vi "Corrupt Frame.vi"(6 "Frame Infos Array":T3[](array[typedef]) {"CRC Index" min=-7 max=7; "DLC Length  Corruption Index" min=-8 max=8}, 8 "error in (no error)":errorcluster, 9 "Engine Run-Time Data Cluster In":T5 {"Compiled Data"."Corruption Info DUT_Network"."Frame Infos Array"."CRC Index" min=-7 max=7; "Compiled Data"."Corruption Info DUT_Network"."Frame Infos Array"."DLC Length  Corruption Index" min=-8 max=8; "Compiled Data"."Corruption Info Network_DUT"."Frame Infos Array"."CRC Index" min=-7 max=7; "Compiled Data"."Corruption Info Network_DUT"."Frame Infos Array"."DLC Length  Corruption Index" min=-8 max=8; "Specified Channel Ref List Out" format="%.0x"; "Specified Channel Ref List In" format="%.0x"}, 10 "Corrupt IDs Array":u32[](array[numeric]), 11 "CAN frame":T1 {"payload" format="%x"; "timestamp" format="%<%.7X\n%x>T"; "type" items=["CAN Data"=0, "CAN Remote"=1, "CAN Bus Error"=2, "CAN 2.0 Data"=8, "CAN FD Data"=16, "CAN FD+BRS Data"=24, "J1939 Data"=192, "Delay"=224, "Log Trigger"=225, "Start Trigger"=226]; "identifier" format="%x"}) -> (0 "error out":errorcluster, 2 "Disable Frame":bool, 3 "Frame Data":T1 {"payload" format="%x"; "timestamp" format="%<%.7X\n%x>T"; "type" items=["CAN Data"=0, "CAN Remote"=1, "CAN Bus Error"=2, "CAN 2.0 Data"=8, "CAN FD Data"=16, "CAN FD+BRS Data"=24, "J1939 Data"=192, "Delay"=224, "Log Trigger"=225, "Start Trigger"=226]; "identifier" format="%x"})   [LabVIEW 2018, in "CAN Gateway Engine.lvlib"]
uses:
  CAN Gateway Engine.lvlib
  <vilib>/xnet/xnet.llb/XNET Frame CAN.ctl
  <vilib>/xnet/xnet.llb/XNET Frame Type CAN.ctl
  Shared/CTLs/Runtime engine Data.ctl
  <vilib>/NI Veristand/Custom Device API/Custom Device Engine Event Ref.ctl
  <vilib>/NI Veristand/Custom Device API/Custom Device Item Ref.ctl
  Shared/CTLs/Compiled Data.ctl
  Shared/CTLs/Corruption Info.ctl
  Shared/CTLs/Frame.ctl
  Shared/CTLs/Signal_Data_Trigger.ctl
  <vilib>/NI Veristand/Custom Device API/Custom Device API.lvlib
  Shared/CAN Gateway Shared.lvlib
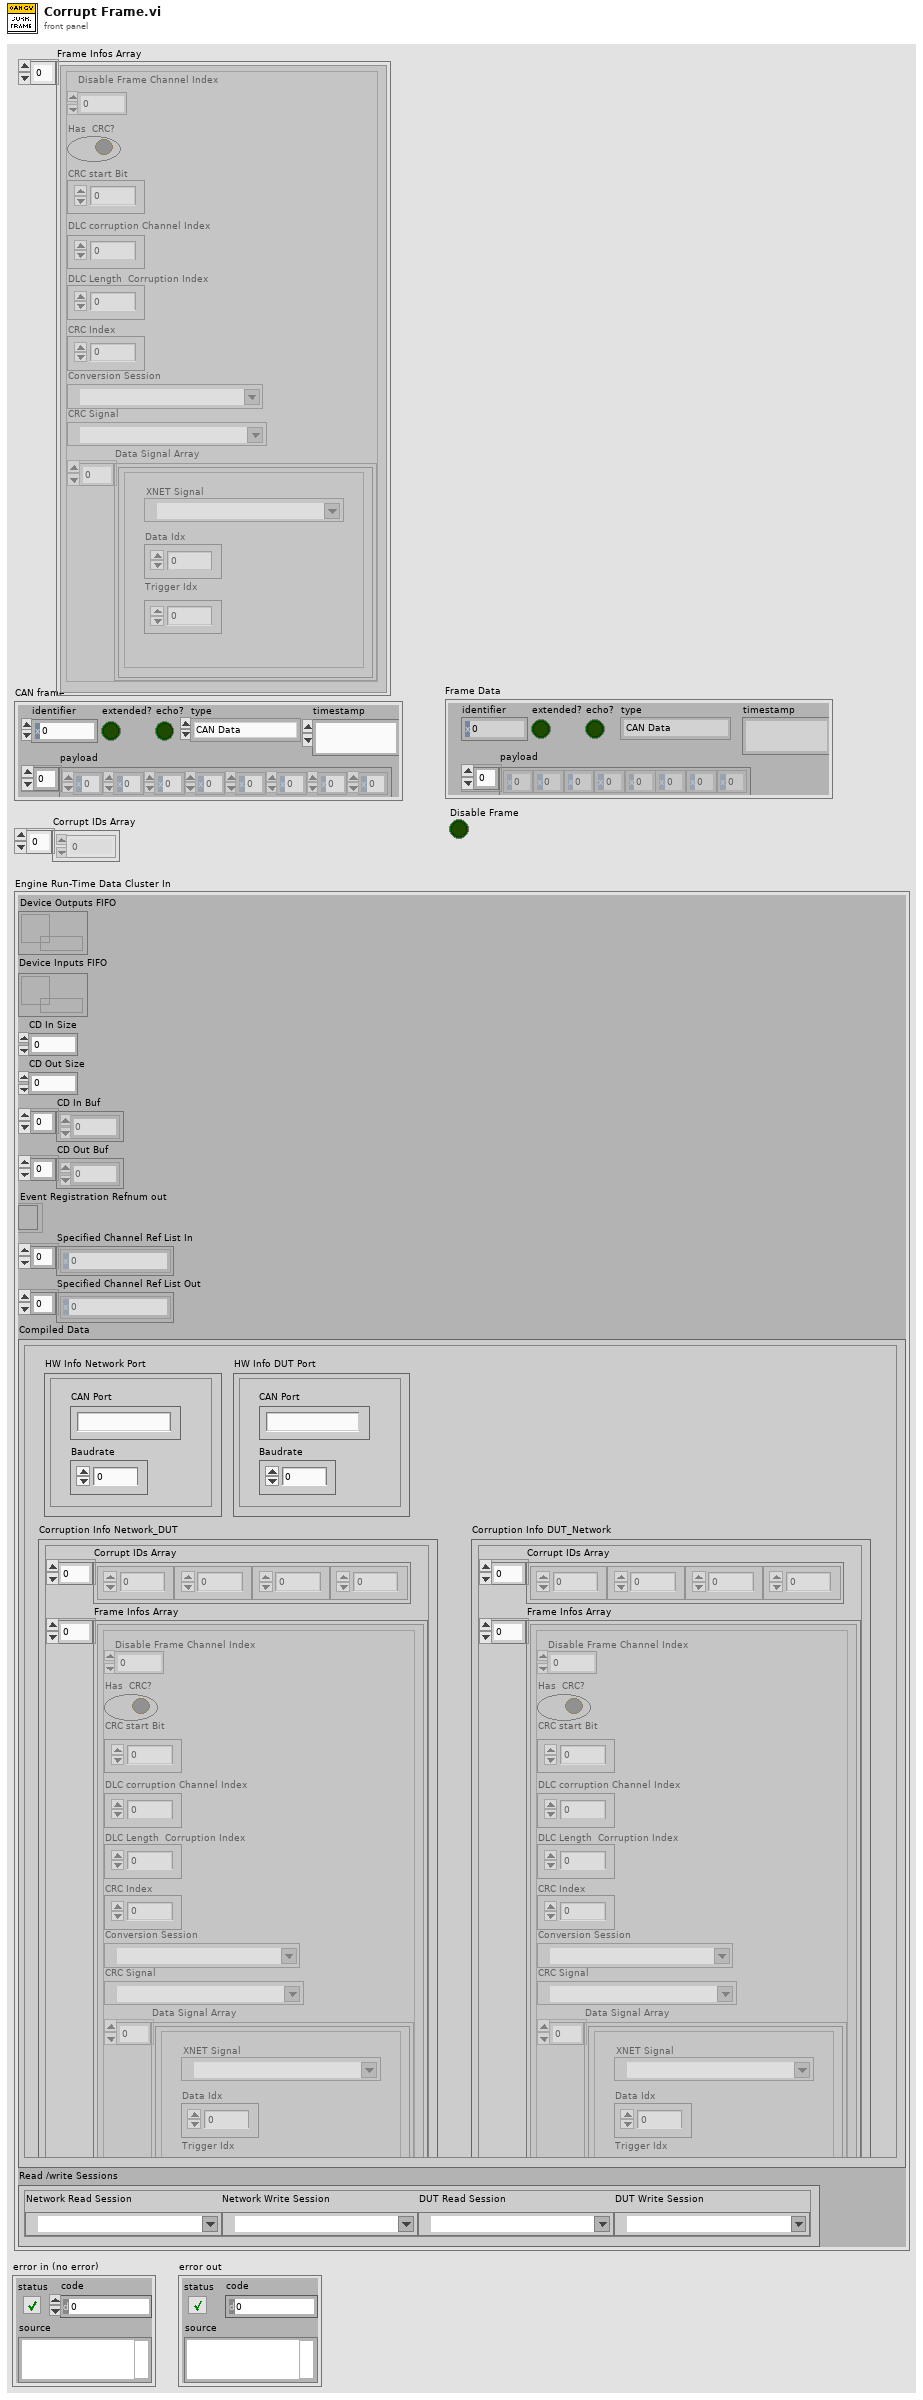
[diagram p1: front panel]
types:
  T1 = typedef "XNET Frame CAN.ctl" = cluster{"timestamp":timestamp, "payload":u8[], "identifier":u32, "type":T2, "extended?":bool, "echo?":bool}
  T2 = typedef "XNET Frame Type CAN.ctl" = u8
  T3 = typedef "CAN Gateway Shared.lvlib/Frame.ctl" = cluster{"Disable Frame Channel Index":i32, "Has  CRC?":bool, "CRC start Bit":u32, "DLC corruption Channel Index":i32, "DLC Length  Corruption Index":i32, "CRC Index":i32, "Conversion Session":refnum<k21>, "CRC Signal":refnum<k21>, "Data Signal Array":T4[]}
  T4 = typedef "CAN Gateway Shared.lvlib/Signal_Data_Trigger.ctl" = cluster{"XNET Signal":refnum<k21>, "Data Idx":u32, "Trigger Idx":u32}
  T5 = typedef "CAN Gateway Engine.lvlib/Runtime engine Data.ctl" = cluster{"Device Outputs FIFO":refnum<k33>, "Device Inputs FIFO":refnum<k33>, "CD In Size":i32, "CD Out Size":i32, "CD In Buf":dbl[], "CD Out Buf":dbl[], "Event Registration Refnum out":T6, "Specified Channel Ref List In":T7[], "Specified Channel Ref List Out":T7[], "Compiled Data":T8, "Read /write Sessions":cluster{"Network Read Session":refnum<k21>, "Network Write Session":refnum<k21>, "DUT Read Session":refnum<k21>, "DUT Write Session":refnum<k21>}}
  T6 = typedef "Custom Device API.lvlib/Custom Device Engine Event Ref.ctl" = refnum<event-registration>
  T7 = typedef "Custom Device API.lvlib/Custom Device Item Ref.ctl" = u64
  T8 = typedef "CAN Gateway Shared.lvlib/Compiled Data.ctl" = cluster{"HW Info Network Port":cluster{"CAN Port":string, "Baudrate":u64}, "HW Info DUT Port":cluster{"CAN Port":string, "Baudrate":u64}, "Corruption Info Network_DUT":T9, "Corruption Info DUT_Network":T9}
  T9 = typedef "CAN Gateway Shared.lvlib/Corruption Info.ctl" = cluster{"Corrupt IDs Array":u32[], "Frame Infos Array":T3[]}
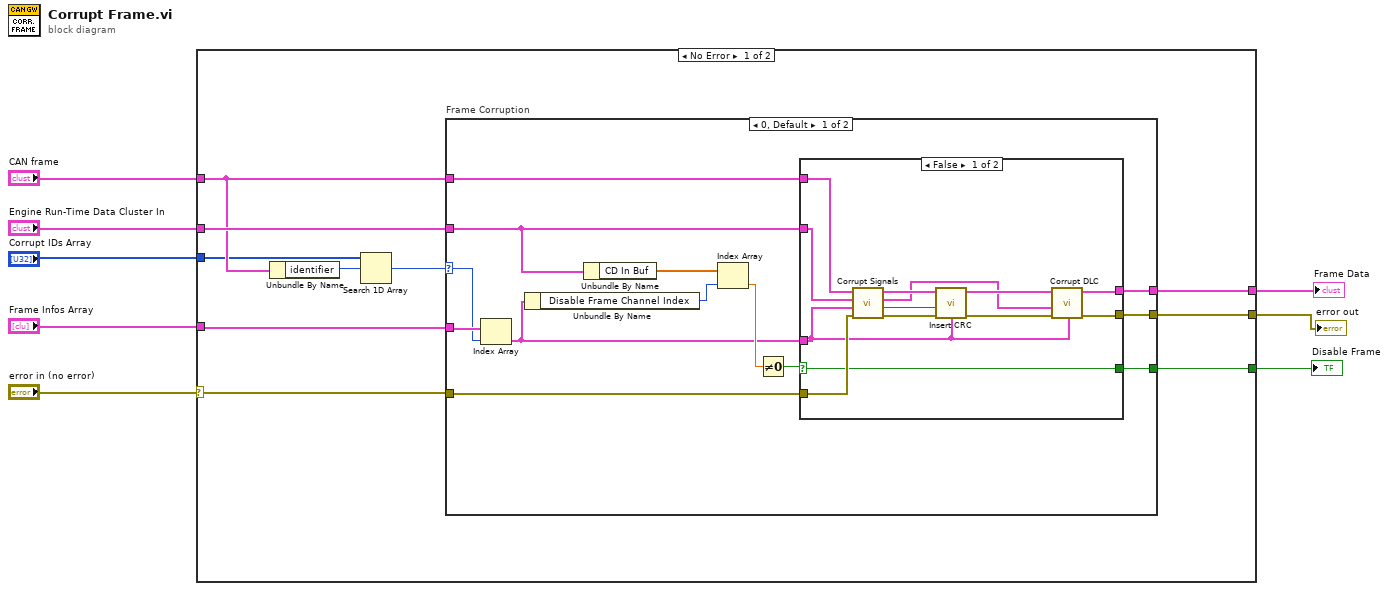
[diagram p0: block diagram]
diagram:
  n1 = case shown="No Error" "error in (no error)" {
    selector: "error in (no error)" -> [w18 w51]
    tunnel: [w17 w51] -> w8
    tunnel: "CAN frame" -> [w12 w50]
    tunnel: "Engine Run-Time Data Cluster In" -> [w15 _]
    tunnel: "Frame Infos Array" -> [w16 _]
    tunnel: "Corrupt IDs Array" -> [w9 _]
    tunnel: [w13 w50] -> w2
    tunnel: [w11 _] -> w1
    frame No Error {
      n2 = Unbundle By Name(w12) -> ("identifier"=w10:u32)
      n3 = Search 1D Array(1D array=w9, element=w10) -> (index of element=w14:i32)  [unwired: 1 in]
      n4 = case "Frame Corruption" shown="0, Default" w14 {
        selector: w14 -> [w30 _]
        tunnel: w12 -> [w29 w48]
        tunnel: w16 -> [w31 _]
        tunnel: w15 -> [w24 _]
        tunnel: w18 -> [w28 w49]
        tunnel: [w26 w49] -> w17
        tunnel: [w27 w48] -> w13
        tunnel: [w25 _] -> w11
        frame 0, Default {
          n5 = Index Array(array=w31, index=w30) -> (element=w19:T3)
          n6 = Unbundle By Name(w19) -> ("Disable Frame Channel Index"=w22:i32)
          n7 = Unbundle By Name(w24) -> ("CD In Buf"=w23:dbl[])
          n8 = Index Array(array=w23, index=w22) -> (element=w20:dbl)
          n9 = Not Equal To 0?(x=w20) -> (x != 0?=w21:bool)
          n10 = case shown="False" w21 {
            selector: w21 -> [w41 w46]
            tunnel: w24 -> [w44 _]
            tunnel: w29 -> [w43 w45]
            tunnel: w28 -> [w42 w47]
            tunnel: [w34 w45] -> w27
            tunnel: [w35 w47] -> w26
            tunnel: w19 -> [w38 _]
            tunnel: [w41 w46] -> w25
            frame False {
              n11 = call "Corrupt Signals.vi"("error in (no error)"=w42, "Frame Infos"=w38, "Engine Run-Time Data Cluster In"=w44, "CAN frame in"=w43) -> ("error out"=w40:errorcluster, "Recalculate CRC?"=w32:bool, "Engine Run-Time Data Cluster Out"=w33:T5, "CAN frame out"=w39:T1)  [unwired: 4 in]
              n12 = call "Insert CRC.vi"("error in (no error)"=w40, "Recalculate CRC?"=w32, "Frame Infos"=w38, "CAN frame in"=w39) -> ("error out"=w36:errorcluster, "CAN frame out"=w37:T1)  [unwired: 6 in]
              n13 = call "Corrupt DLC.vi"("error in (no error)"=w36, "Engine Run-Time Data Cluster In"=w33, "Frame Infos"=w38, "CAN frame in"=w37) -> ("error out"=w35:errorcluster, "CAN frame out"=w34:T1)  [unwired: 6 in]
            }
            frame True {
            }
          }
        }
        frame -1 {
        }
      }
    }
    frame Error {
    }
  }
  "error out" <- w8
  "Frame Data" <- w2
  "Disable Frame" <- w1
